vi "ma_Spectrum Peak Hold no State.vi"(6 "state info":T2 {"real spectrum" format="%0.2f"; "averages completed" format="%0.2f"; "df" format="%0.2f"; "complex spectrum" format="%0.2f"; "spectrum parameters"."window" items=["Rectangle"=0, "Hanning"=1, "Hamming"=2, "Blackman-Harris"=3, "Exact Blackman"=4, "Blackman"=5, "Flat Top"=6, "4 Term B-Harris "=7, "7 Term B-Harris"=8, "Low Sidelobe"=9, "Blackman Nuttall"=11, "Triangle"=30, "Bartlett-Hanning"=31, "Bohman"=32, "Parzen"=33, "Welch"=34, "Kaiser"=60, "Dolph-Chebyshev"=61, "Gaussian"=62]; "dt" format="%0.2f"; "timestamp" format="%0.2f"; "dt history" format="%0.2f"; "t0 history" format="%0.2f"}, 8 "restart averaging (F)":bool, 9 "averaging parameters":T3={"averaging mode"=enum."No averaging", "weighting mode"=enum."Exponential", "number of averages"=10} {"number of averages" min=1}, 11 "real spectrum":dbl[](array[numeric]) format="%0.2f") -> (0 "averages completed":dbl format="%0.2f", 1 "averaging done":bool, 3 "peak spectrum":dbl[](array[numeric]) format="%0.2f", 4 "state info":T2 {"real spectrum" format="%0.2f"; "averages completed" format="%0.2f"; "df" format="%0.2f"; "complex spectrum" format="%0.2f"; "spectrum parameters"."window" items=["Rectangle"=0, "Hanning"=1, "Hamming"=2, "Blackman-Harris"=3, "Exact Blackman"=4, "Blackman"=5, "Flat Top"=6, "4 Term B-Harris "=7, "7 Term B-Harris"=8, "Low Sidelobe"=9, "Blackman Nuttall"=11, "Triangle"=30, "Bartlett-Hanning"=31, "Bohman"=32, "Parzen"=33, "Welch"=34, "Kaiser"=60, "Dolph-Chebyshev"=61, "Gaussian"=62]; "dt" format="%0.2f"; "timestamp" format="%0.2f"; "dt history" format="%0.2f"; "t0 history" format="%0.2f"})   [LabVIEW 2020, in "NI_MAPro.lvlib"]
uses:
  NI_MAPro.lvlib
  windowTd.ctl
  NI_AALPro.lvlib
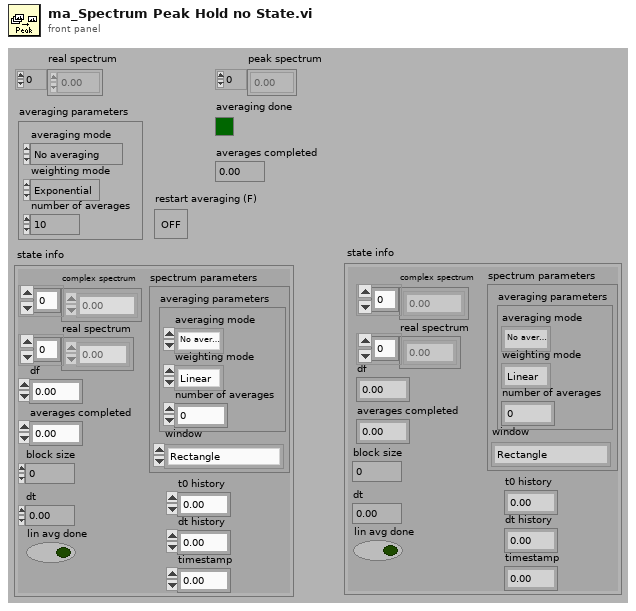
[diagram p1: front panel]
types:
  T1 = typedef "NI_AALPro.lvlib/windowTd.ctl" = u32
  T2 = cluster{"block size":i32, "dt":dbl, "spectrum parameters":cluster{"averaging parameters":cluster{"averaging mode":enum16{"No averaging", "Vector averaging", "RMS averaging", "Peak hold"}, "weighting mode":enum16{"Linear", "Exponential"}, "number of averages":u32}, "window":T1}, "df":dbl, "averages completed":dbl, "complex spectrum":cdb[], "real spectrum":dbl[], "t0 history":dbl, "dt history":dbl, "timestamp":dbl, "lin avg done":bool}
  T3 = cluster{"averaging mode":enum16{"No averaging", "Vector averaging", "RMS averaging", "Peak hold"}, "weighting mode":enum16{"Linear", "Exponential"}, "number of averages":u32}
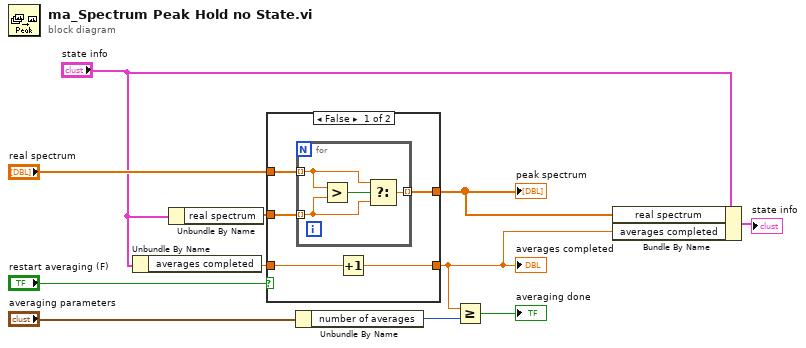
[diagram p0: block diagram]
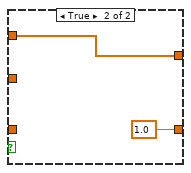
[diagram p2: hidden frame]
diagram:
  n1 = Unbundle By Name("state info") -> ("averages completed"=w1:dbl)
  n2 = Unbundle By Name("state info") -> ("real spectrum"=w2:dbl[])
  n3 = case shown="False" "restart averaging (F)" {
    tunnel: [w12 w21] -> w6
    tunnel: [w15 1.0] -> w7
    tunnel: w1 -> [w16 _]
    tunnel: w2 -> [w13 _]
    tunnel: "real spectrum" -> [w14 w21]
    frame False {
      n4 = for {
        tunnel: w14 -> [w19] mode=indexing
        tunnel: w13 -> [w18] mode=indexing
        tunnel: [w17] -> w12 mode=indexing
        n5 = Greater?(x=w19, y=w18) -> (0:w20:bool)
        n6 = Select(t=w19, s=w20, f=w18) -> (s? t:f=w17:dbl)
      }
      n7 = Increment(x=w16) -> (x+1=w15:dbl)
    }
    frame True {
    }
  }
  "peak spectrum" <- w6
  "averages completed" <- w7
  n8 = Unbundle By Name("averaging parameters") -> ("number of averages"=w3:u32)
  n9 = Greater Or Equal?(x=w7, y=w3) -> (x >= y?=→"averaging done":bool)
  n10 = Bundle By Name(cluster="state info", "real spectrum"=w6, "averages completed"=w7) -> (→"state info":T2)
